vi "Get Value at Path Array.vi"(0 "Variant in":variant, 2 "Path in":string[](array[string]), 11 "error in (no error)":errorcluster) -> (4 "Variant out":variant, 8 "Element out":variant, 15 "error out":errorcluster)   [LabVIEW 2017, in "Advanced Variant Tools.lvlib"]
uses:
  Advanced Variant Tools.lvlib
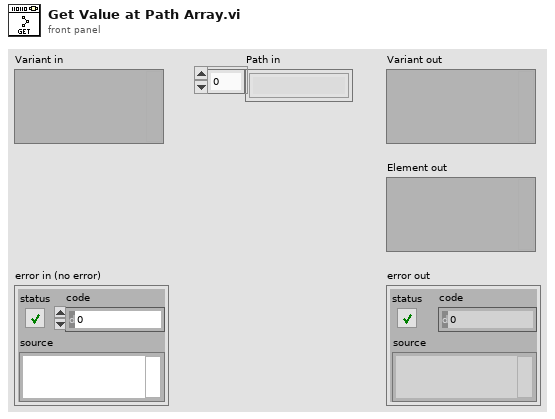
[diagram p1: front panel]
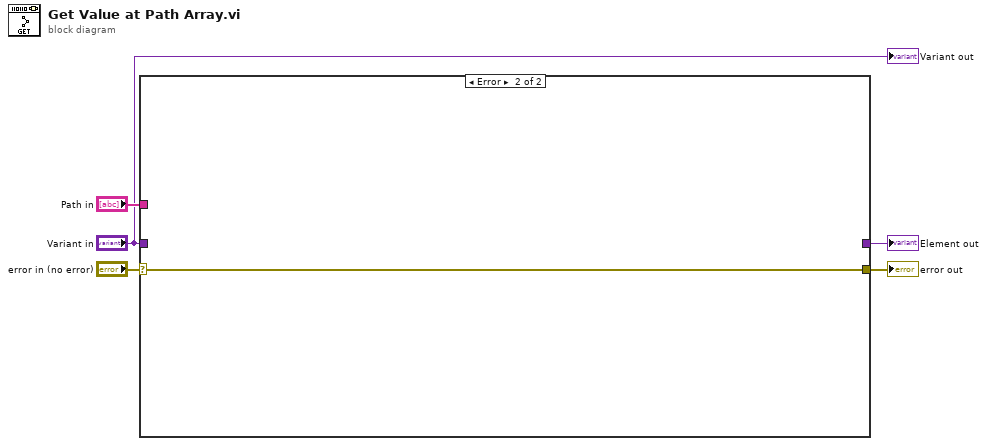
[diagram p0: block diagram]
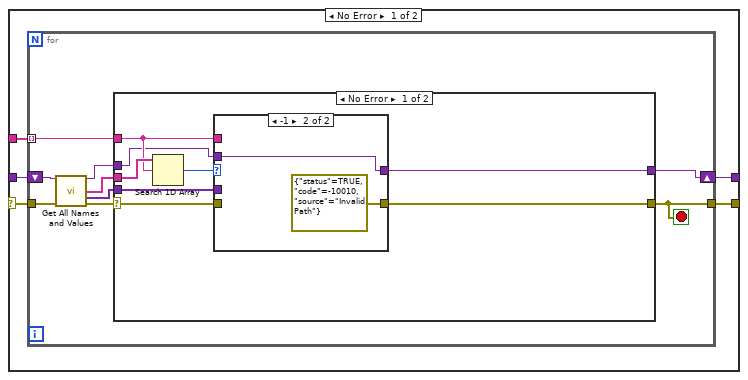
[diagram p2: hidden frame]
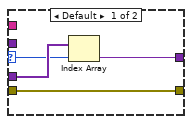
[diagram p3: hidden frame]
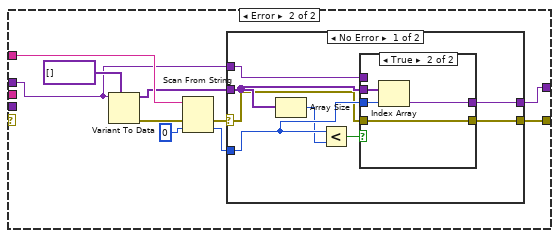
[diagram p4: hidden frame]
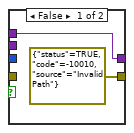
[diagram p5: hidden frame]
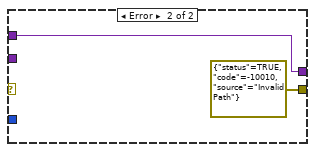
[diagram p6: hidden frame]
diagram:
  n1 = case shown="Error" "error in (no error)" {
    selector: "error in (no error)" -> [w6 w60]
    tunnel: "Path in" -> [w10 _]
    tunnel: "Variant in" -> [w9 _]
    tunnel: [w8 _] -> w3
    tunnel: [w7 w60] -> w2
    frame No Error {
      n2 = for {
        tunnel: w10 -> [w15] mode=indexing
        shift-right: [w19] -> w8
        shift-left: w9 -> [w18]
        tunnel: [w17] -> w7
        tunnel: w6 -> [w13]
        stop <- w17 stop-if-true
        n3 = call "Get All Names and Values.vi"("Variant (Cluster) In"=w18, "error in"=w13) -> ("Variant (Cluster) Out"=w16:variant, "Element Names"=w12:string[], "Values"=w11:variant[], "error out"=w14:errorcluster)  [unwired: 9 in, 1 out]
        n4 = case shown="No Error" w14 {
          selector: w14 -> [w22 _]
          tunnel: [w23 w38] -> w19
          tunnel: [w25 w43] -> w17
          tunnel: w16 -> [w20 w34]
          tunnel: w15 -> [w21 w42]
          tunnel: w12 -> [w27 _]
          tunnel: w11 -> [w24 _]
          frame No Error {
            n5 = Search 1D Array(1D array=w27, element=w21) -> (index of element=w26:i32)  [unwired: 1 in]
            n6 = case shown="-1" w26 {
              selector: w26 -> [w30 _]
              tunnel: [w28 errorcluster {"status"=TRUE, "code"=-10010, "source"="Invalid Path"} ("error IO")] -> w25
              tunnel: w24 -> [w31 _]
              tunnel: [w29 w32] -> w23
              tunnel: w22 -> [w28 _]
              tunnel: w21 -> [_ _]
              tunnel: w20 -> [_ w32]
              frame Default {
                n7 = Index Array(array=w31, index=w30) -> (element=w29:variant)
              }
              frame -1 {
              }
            }
          }
          frame Error {
            n8 = Variant To Data(type=variant[] [], Variant=w34) -> (data=w36:variant[], error out=w35:errorcluster)  [unwired: 1 in]
            n9 = Scan From String(input string=w42, error in=w35, default 1=0 ("default value 1")) -> (error out=w40:errorcluster, output 1=w39:i32)  [unwired: 2 in, 2 out]
            n10 = case shown="No Error" w40 {
              selector: w40 -> [w45 _]
              tunnel: [w46 errorcluster {"status"=TRUE, "code"=-10010, "source"="Invalid Path"} ("error IO")] -> w43
              tunnel: w39 -> [w49 _]
              tunnel: w36 -> [w50 _]
              tunnel: [w51 w58] -> w38
              tunnel: w34 -> [w44 w58]
              frame No Error {
                n11 = Array Size(array=w50) -> (size(s)=w48:i32)
                n12 = Less?(x=w49, y=w48) -> (x < y?=w47:bool)
                n13 = case shown="True" w47 {
                  tunnel: [w52 w57] -> w51
                  tunnel: w50 -> [_ w56]
                  tunnel: w49 -> [_ w55]
                  tunnel: [errorcluster {"status"=TRUE, "code"=-10010, "source"="Invalid Path"} ("error IO") w54] -> w46
                  tunnel: w45 -> [_ w54]
                  tunnel: w44 -> [w52 _]
                  frame False {
                  }
                  frame True {
                    n14 = Index Array(array=w56, index=w55) -> (element=w57:variant)
                  }
                }
              }
              frame Error {
              }
            }
          }
        }
      }
    }
    frame Error {
    }
  }
  "error out" <- w2
  "Element out" <- w3
  "Variant out" <- "Variant in"
